vi "Handshake.vi"(8 "error in":errorcluster, 11 "RawSocket Handler in":refnum<class "RawSocket TCP Handler.lvclass">) -> (0 "error out":errorcluster, 3 "RawSocket Handler out":refnum<class "RawSocket TCP Handler.lvclass">)   [LabVIEW 2020, in "wamplv.lvlib" / "RawSocket TCP Handler.lvclass"]
uses:
  RawSocket TCP Handler.lvclass
  TypeDefs/Serilisation Types.ctl
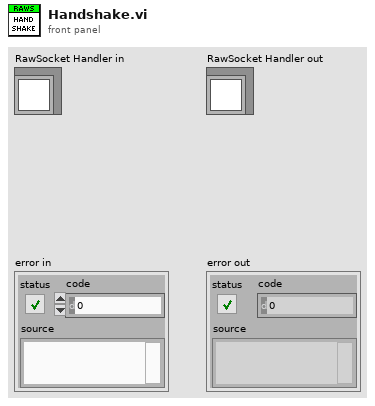
[diagram p1: front panel]
types:
  T1 = typedef "wamplv.lvlib/RawSocket TCP Handler.lvclass/Serilisation Types.ctl" = u8
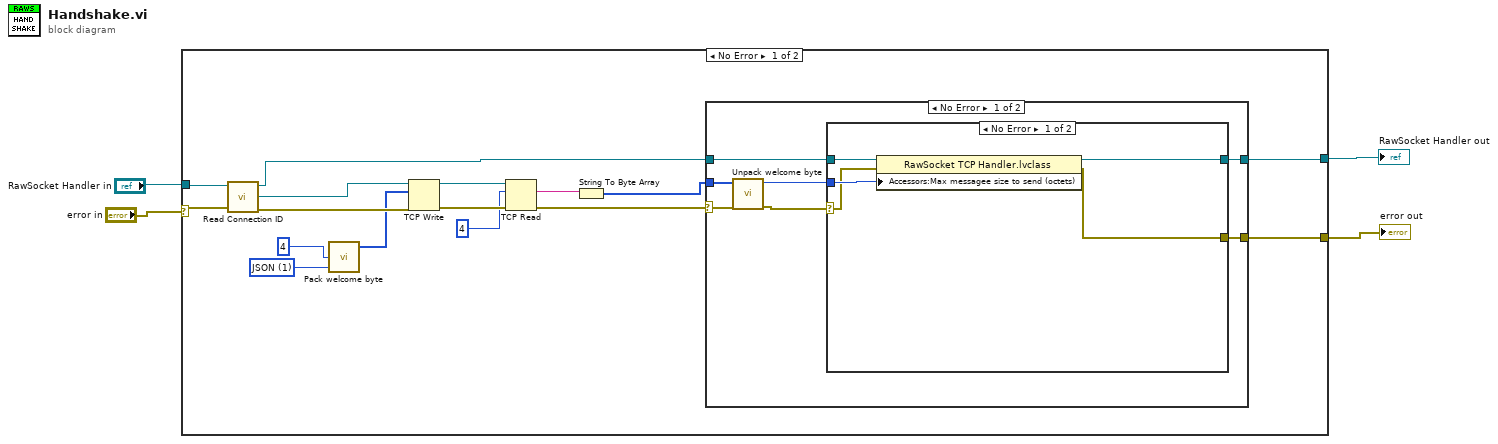
[diagram p0: block diagram]
diagram:
  n1 = case shown="No Error" "error in" {
    selector: "error in" -> [w19 w38]
    tunnel: [w5 w38] -> w3
    tunnel: [w6 w37] -> w4
    tunnel: "RawSocket Handler in" -> [w20 w37]
    frame No Error {
      w15 = T1 1 items=["JSON"=1, "MessagePack"=2] ("Serliaser")
      n2 = call-dynamic "Read Connection ID.vi"("error in (no error)"=w19, "RawSocket Handler in"=w20) -> ("error out"=w17:errorcluster, "Connection ID"=w18:refnum<k5>, "RawSocket Handler out"=w13:refnum<class "RawSocket TCP Handler.lvclass">)  [unwired: 7 in]
      n3 = call "Pack welcome byte.vi"("Serliaser"=w15, "Length (octets)"=u8 4) -> ("Bytes"=w14:u8[])  [unwired: 3 in]
      n4 = TCP Write(connection ID=w18, data in=w14, error in (no error)=w17) -> (connection ID out=w12:refnum<k5>, error out=w11:errorcluster)  [unwired: 1 in, 1 out]
      n5 = TCP Read(connection ID=w12, bytes to read=4, error in (no error)=w11) -> (data out=w10:string, error out=w8:errorcluster)  [unwired: 2 in, 1 out]
      n6 = String To Byte Array(string=w10) -> (unsigned byte array=w9:u8[])
      n7 = case shown="No Error" w8 {
        selector: w8 -> [w27 w36]
        tunnel: w9 -> [w25 _]
        tunnel: w13 -> [w23 w35]
        tunnel: [w22 w35] -> w6
        tunnel: [w21 w36] -> w5
        frame No Error {
          n8 = call "Unpack welcome byte.vi"("error in"=w27, "Byte"=w25) -> ("error (out)"=w26:errorcluster, "Length (octets)"=w24:u8)  [unwired: 7 in, 1 out]
          n9 = case shown="No Error" w26 {
            selector: w26 -> [w29 w34]
            tunnel: w24 -> [w32 _]
            tunnel: w23 -> [w31 w33]
            tunnel: [w30 w33] -> w22
            tunnel: [w28 w34] -> w21
            frame No Error {
              n10 = property class="RawSocket TCP Handler.lvclass"(reference=w31, error in=w29, "Accessors:Max messagee size to send (octets)"=w32) -> (reference out=w30:refnum<class "RawSocket TCP Handler.lvclass">, error out=w28:errorcluster)
            }
            frame Error {
            }
          }
        }
        frame Error {
        }
      }
    }
    frame Error {
    }
  }
  "RawSocket Handler out" <- w4
  "error out" <- w3
